vi "test-GetLvClassXXX.vi"() -> ()   [LabVIEW 2019]
uses:
  LabVIEW-ProviderShell/Example3/Provider/ProviderClass.lvclass
  28aaa983-7d96-4935-8716-11887d24da21.vi
  b8ff2e94-8cac-457e-a4d3-2d7f87fd7446.vi
  1eda3c33-e1b6-4196-853d-418c18817bb0.vi
  558217e8-0e25-4930-b1dd-1805d4fdfc38.vi
  8724bd50-1a80-4828-a56e-1d157abe3a21.vi
  0644aedd-2a43-4a3b-98fd-516f9be53c0f.vi
  18f549e6-cfa8-4a34-bc90-2f692c9cb377.vi
  <vilib>/Utility/error.llb/Clear Errors.vi
  <userlib>/NEVSTOP-Programming-Palette/String/Strip Class Function Name_nevstop.vi
  28aaa983-7d96-4935-8716-11887d24da21.vi/ac4ff739-4ca7-446b-9cae-3ed43b506181.vi
  28aaa983-7d96-4935-8716-11887d24da21.vi/810ca34f-2919-4602-a96f-2f6eb403073d.vi
  b8ff2e94-8cac-457e-a4d3-2d7f87fd7446.vi/5c9830ef-78ea-4d05-95d4-934bfe8ea8ca.vi
  1eda3c33-e1b6-4196-853d-418c18817bb0.vi/13321162-f811-47ed-b28f-96d2257e91d5.vi
  1eda3c33-e1b6-4196-853d-418c18817bb0.vi/359622d5-4a99-4feb-a4b8-751b4f753a0c.vi
  558217e8-0e25-4930-b1dd-1805d4fdfc38.vi/4837e199-d753-4b5a-aac5-380a7c9b0d3d.vi
  558217e8-0e25-4930-b1dd-1805d4fdfc38.vi/9eeb00ff-2a49-4b01-b565-495446fab940.vi
  8724bd50-1a80-4828-a56e-1d157abe3a21.vi/c21344a8-6eba-4e58-9dd2-35e92eb98815.vi
  0644aedd-2a43-4a3b-98fd-516f9be53c0f.vi/0b25f828-9ccf-4482-ba3a-9f3a69078ca7.vi
  0644aedd-2a43-4a3b-98fd-516f9be53c0f.vi/03c2ae9d-d2d5-4de2-9314-e60834a694d9.vi
panel:
  out "lv-providershell-example3.lvlib:ProviderClass.lvclass":refnum<class "ProviderClass.lvclass">
  out "class name":string
  out "ParentName 2":string
  out "Version 2":T1
  out "Array 2":string[](array[string])
  out "Array":string[](array[string])
  out "Version":T1
  out "ParentName":string
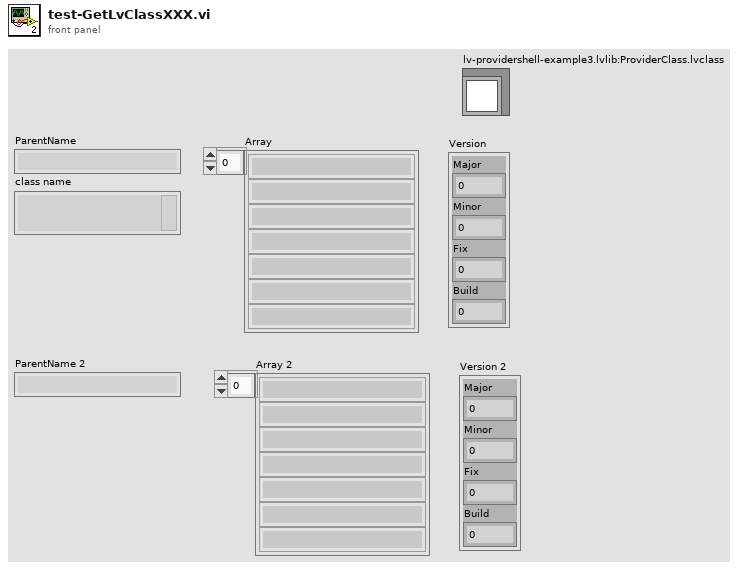
[diagram p1: front panel]
types:
  T1 = cluster{"Major":u16, "Minor":u16, "Fix":u16, "Build":u16}
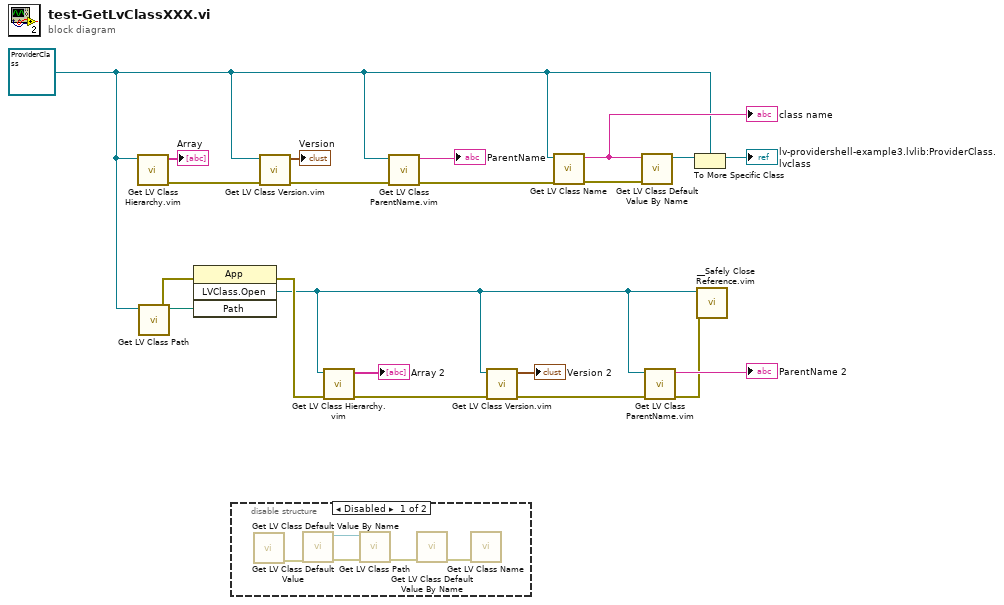
[diagram p0: block diagram]
diagram:
  w1 = refnum<class "ProviderClass.lvclass"> refnum ("lv-providershell-example3.lvlib:ProviderClass.lvclass")
  n1 = call "Get LV Class Hierarchy.vim"("LvObject(Class/ClassRefnum)"=w1) -> ("error in (no error) (dup)"=w21:errorcluster, "Array"=→"Array":string[])  [unwired: 9 in]
  n2 = call <vilib>:"Get LV Class Path.vi"("object"=w1) -> ("error out"=w16:errorcluster, "class path"=w15:path)  [unwired: 9 in]
  n3 = invoke on="Invoke Node" class="App" method="LVClass.Open"(error in=w16, "Path"=w15) -> (error out=w8:errorcluster, "LVClass.Open"=w2:refnum<vi>)  [unwired: 2 in, 2 out]
  n4 = disable-structure "Diagram Disable Structure" shown="Disabled" {
    frame Disabled {
      n5 = call <vilib>:"Get LV Class Default Value By Name.vi"() -> ("error out"=w22:errorcluster)  [unwired: 10 in, 1 out]
      n6 = call <vilib>:"Get LV Class Default Value.vi"("error in (no error)"=w22) -> ("error out"=w26:errorcluster, "object"=w25:refnum<class>)  [unwired: 9 in]
      n7 = call <vilib>:"Get LV Class Path.vi"("error in (no error)"=w26, "object"=w25) -> ("error out"=w24:errorcluster)  [unwired: 8 in, 1 out]
      n8 = call <vilib>:"Get LV Class Default Value By Name.vi"("error in (no error)"=w24) -> ("error out"=w23:errorcluster)  [unwired: 9 in, 1 out]
      n9 = call <vilib>:"Get LV Class Name.vi"("error in (no error)"=w23) -> ()  [unwired: 9 in, 2 out]
    }
    frame Enabled {
    }
  }
  n10 = call "Get LV Class Version.vim"("error in (no error)"=w21, "LvObject"=w1) -> ("error in (no error) (dup)"=w20:errorcluster, "Version"=→"Version":T1)  [unwired: 8 in]
  n11 = call "Get LV Class Hierarchy.vim"("error in (no error)"=w8, "LvObject(Class/ClassRefnum)"=w2) -> ("error in (no error) (dup)"=w10:errorcluster, "Array"=→"Array 2":string[])  [unwired: 8 in]
  n12 = call "Get LV Class ParentName.vim"("error in (no error)"=w20, "LvObject"=w1) -> ("error in (no error) (dup)"=w7:errorcluster, "ParentName"=→"ParentName":string)  [unwired: 8 in]
  n13 = call "Get LV Class Version.vim"("error in (no error)"=w10, "LvObject"=w2) -> ("error in (no error) (dup)"=w11:errorcluster, "Version"=→"Version 2":T1)  [unwired: 8 in]
  n14 = call <vilib>:"Get LV Class Name.vi"("error in (no error)"=w7, "object"=w1) -> ("error out"=w6:errorcluster, "class name"=w5:string)  [unwired: 8 in]
  "class name" <- w5
  n15 = call <vilib>:"Get LV Class Default Value By Name.vi"("error in (no error)"=w6, "class name"=w5) -> ("object"=w4:refnum<class>)  [unwired: 8 in, 1 out]
  n16 = call "Get LV Class ParentName.vim"("error in (no error)"=w11, "LvObject"=w2) -> ("error in (no error) (dup)"=w9:errorcluster, "ParentName"=→"ParentName 2":string)  [unwired: 8 in]
  n17 = To More Specific Class(target class=w1, reference=w4) -> (specific class reference=→"lv-providershell-example3.lvlib:ProviderClass.lvclass":refnum<class "ProviderClass.lvclass">)  [unwired: 1 in, 1 out]
  n18 = call "__Safely Close Reference.vim"("error in (no error)"=w9, "LVClassLibrary in"=w2) -> ()  [unwired: 9 in, 1 out]
